vi "TLB Native Dynamic Events ver 0.05.vi"() -> ()   [LabVIEW 2018]
uses:
  Labview Training Phase 2/Enum Controls/States for Action Engine.ctl
  Type def/TLB event states.ctl
  Type def/TLB MHL States.ctl
  <vilib>/Studica/Studica Toolkit/Background/I2C Channel.ctl
  <vilib>/Studica/Studica Toolkit/NavX/NavX.lvlib
  <vilib>/myRIO/Common/Instrument Driver Framework/myRIO v1.0/AI/typedefs/AI Channels Enum.ctl
  <vilib>/myRIO/Common/Instrument Driver Framework/myRIO v1.0/AI/typedefs/AI Channels List.ctl
  <vilib>/Studica/Studica Toolkit/Background/Mxp Selection.ctl
  <vilib>/ptbypt/NI_PtbyPt.lvlib
panel:
  out "Yaw":dbl
  in  "NavX Zero Yaw":bool
  out "NavX Info Out":T2
  out "LinearAcceleration":T3
  out "Displacement":T4
  out "YRPHfH":T5
  in  "y":dbl=-1.2 format="%#_13g"
  out "Distance":T6
  in  "Return to IDLE":bool
  out "Sharp IR Distance":dbl
  out "Sharp IR Distance 2":dbl
  out "CM":fxp<+,64,16>
  out "Ultrasonic sensor":dbl format="%0.2f"
  out "Waveform Chart 3":dbl(graph)
  in  "xTargetSpeed":dbl
  in  "yTargetSpeed":dbl
  in  "wTargetSpeed":dbl
  out "Speed":T7
  in  "Reset Encoder 0":bool
  out "Action Queue Items":i32
  out "State Logic Queue Items":i32
  out "Action Queues items":string[](array[string])=["Hardware reset", "Software reset", ""]
  out "State logic":T8=enum."Task 2"
  out "Action State":string
  in  "Tasks Selector":string(combo)="Task 2"
  in  "Stop Queue":bool
  in  "Start Task":bool
  # "Test Programme written by Calvin Loke    Dated: 28 Aug 2019\nTest Programme revised by Dr Alex See   Dated 30 Aug 2019\n\nProgramme version:   TLB Native Dynamic Events ver 0.04b.vi"
  # "System Health Status Update"
  # "Sequence of Actions"
  # "Continuous (Repeated)"
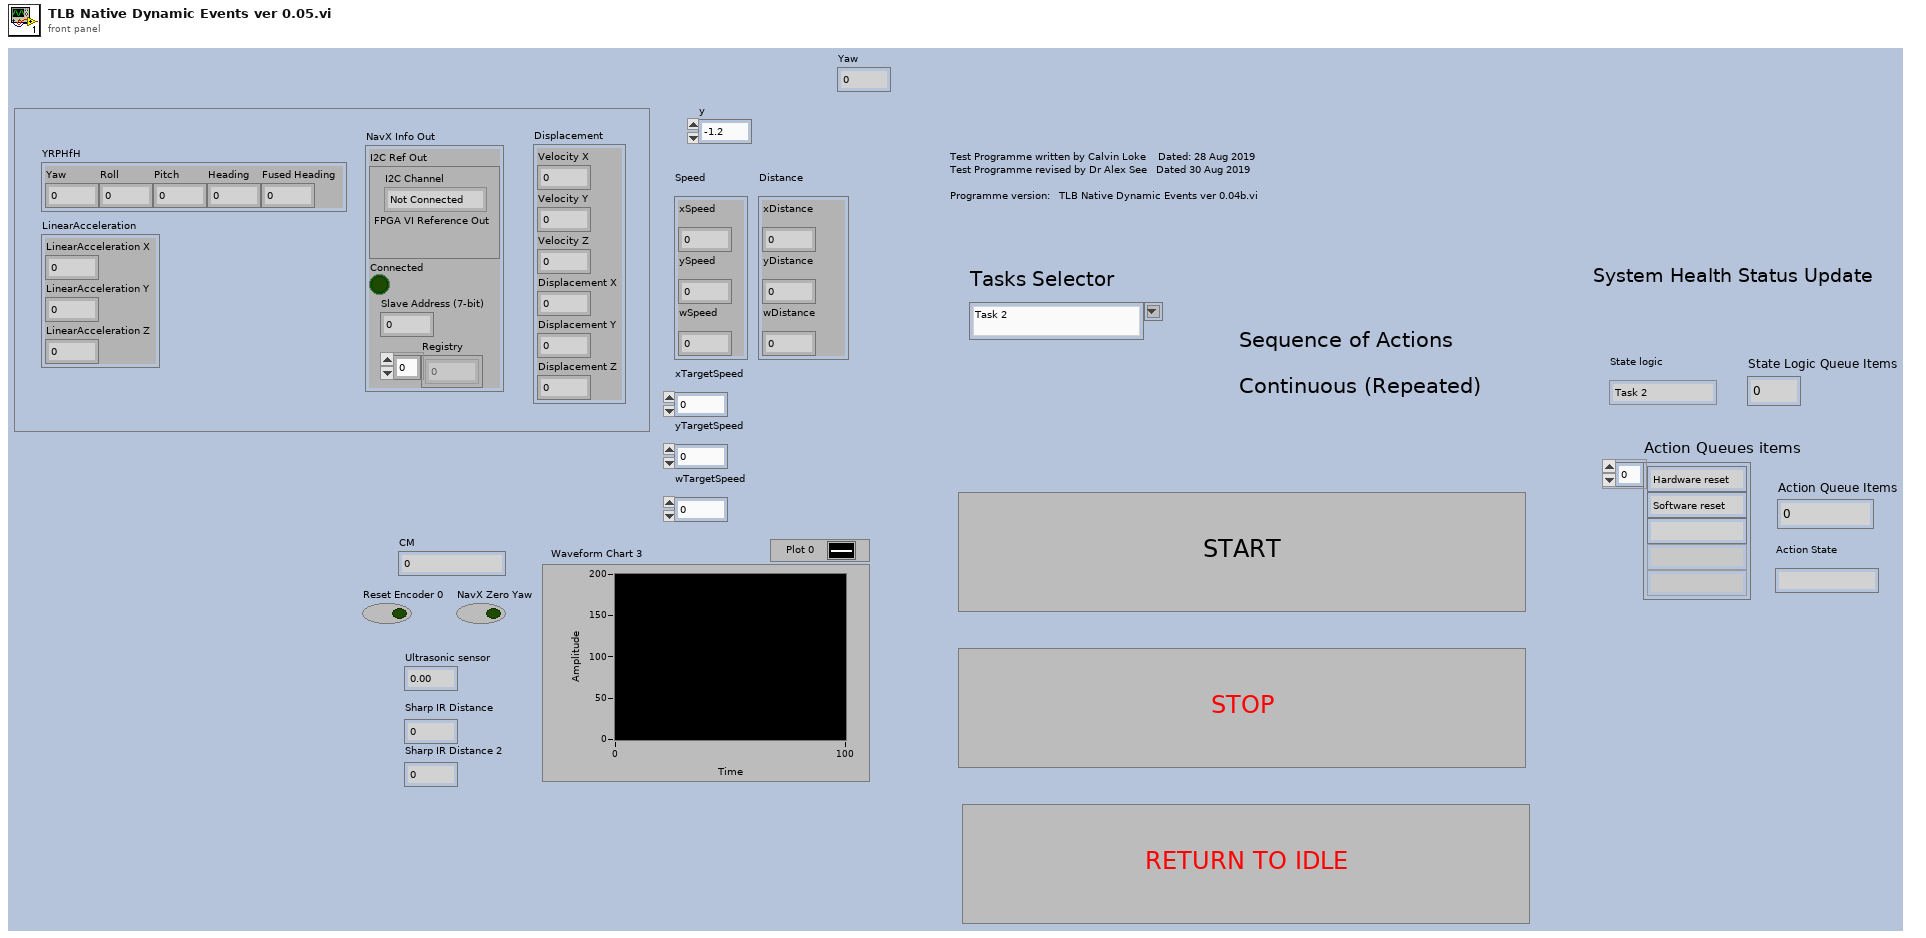
[diagram p1: front panel]
types:
  T1 = typedef "I2C Channel.ctl" = enum16{"Not Connected", "A", "B"}
  T2 = cluster{"I2C Ref Out":cluster{"I2C Channel":T1, "FPGA VI Reference Out":refnum<k20>}, "Connected":bool, "Slave Address (7-bit)":u8, "Registry":u8[]}
  T3 = cluster{"LinearAcceleration X":dbl, "LinearAcceleration Y":dbl, "LinearAcceleration Z":dbl}
  T4 = cluster{"Velocity X":dbl, "Velocity Y":dbl, "Velocity Z":dbl, "Displacement X":dbl, "Displacement Y":dbl, "Displacement Z":dbl}
  T5 = cluster{"Yaw":dbl, "Roll":dbl, "Pitch":dbl, "Heading":dbl, "Fused Heading":dbl}
  T6 = cluster{"xDistance":dbl, "yDistance":dbl, "wDistance":dbl}
  T7 = cluster{"xSpeed":dbl, "ySpeed":dbl, "wSpeed":dbl}
  T8 = typedef "TLB MHL States.ctl" = enum16{"None", "Startup", "Idle", "Processing", "Shutdown", "Reset", "Task 1", "Task 2", "Task 3", "Task 4", "Task 4a", "Task 4b", "Task 4c", "Task 4d", "Task 4e", "Task 4f", "Task 4g", "Task 4h", "Acquire image", "Wall follow mode", "Autodrive", "Autodrive a"}
  T9 = typedef "States for Action Engine.ctl" = enum16{"Initialize", "Write", "Read"}
  T10 = typedef "TLB event states.ctl" = enum16{"Start Sequence", "Exit", "Start Task 1", "Start Task 2", "Start Task 3", "Start Task 4", "Camera vision", "Wall follow mode", "Idle", "Start Drive Straight"}
  T11 = typedef "Mxp Selection.ctl" = enum16{"MXP A", "MXP B"}
  T12 = typedef "AI Channels List.ctl" = T13[]
  T13 = typedef "AI Channels Enum.ctl" = enum16{"Not Connected", "AudioIn/Left", "AudioIn/Right", "C/AI0", "C/AI1", "A/AI0", "A/AI1", "A/AI2", "A/AI3", "A/AI4", "A/AI5", "A/AI6", "A/AI7", "B/AI0", "B/AI1", "B/AI2", "B/AI3", "B/AI4", "B/AI5", "B/AI6", "B/AI7", "AI/AI0", "AI/AI1", "AI/AI2", "AI/AI3", "A/AI0 (DIFF)", "A/AI1 (DIFF)", "A/AI2 (DIFF)", "A/AI3 (DIFF)", "B/AI0 (DIFF)", "B/AI1 (DIFF)", "B/AI2 (DIFF)", "B/AI3 (DIFF)"}
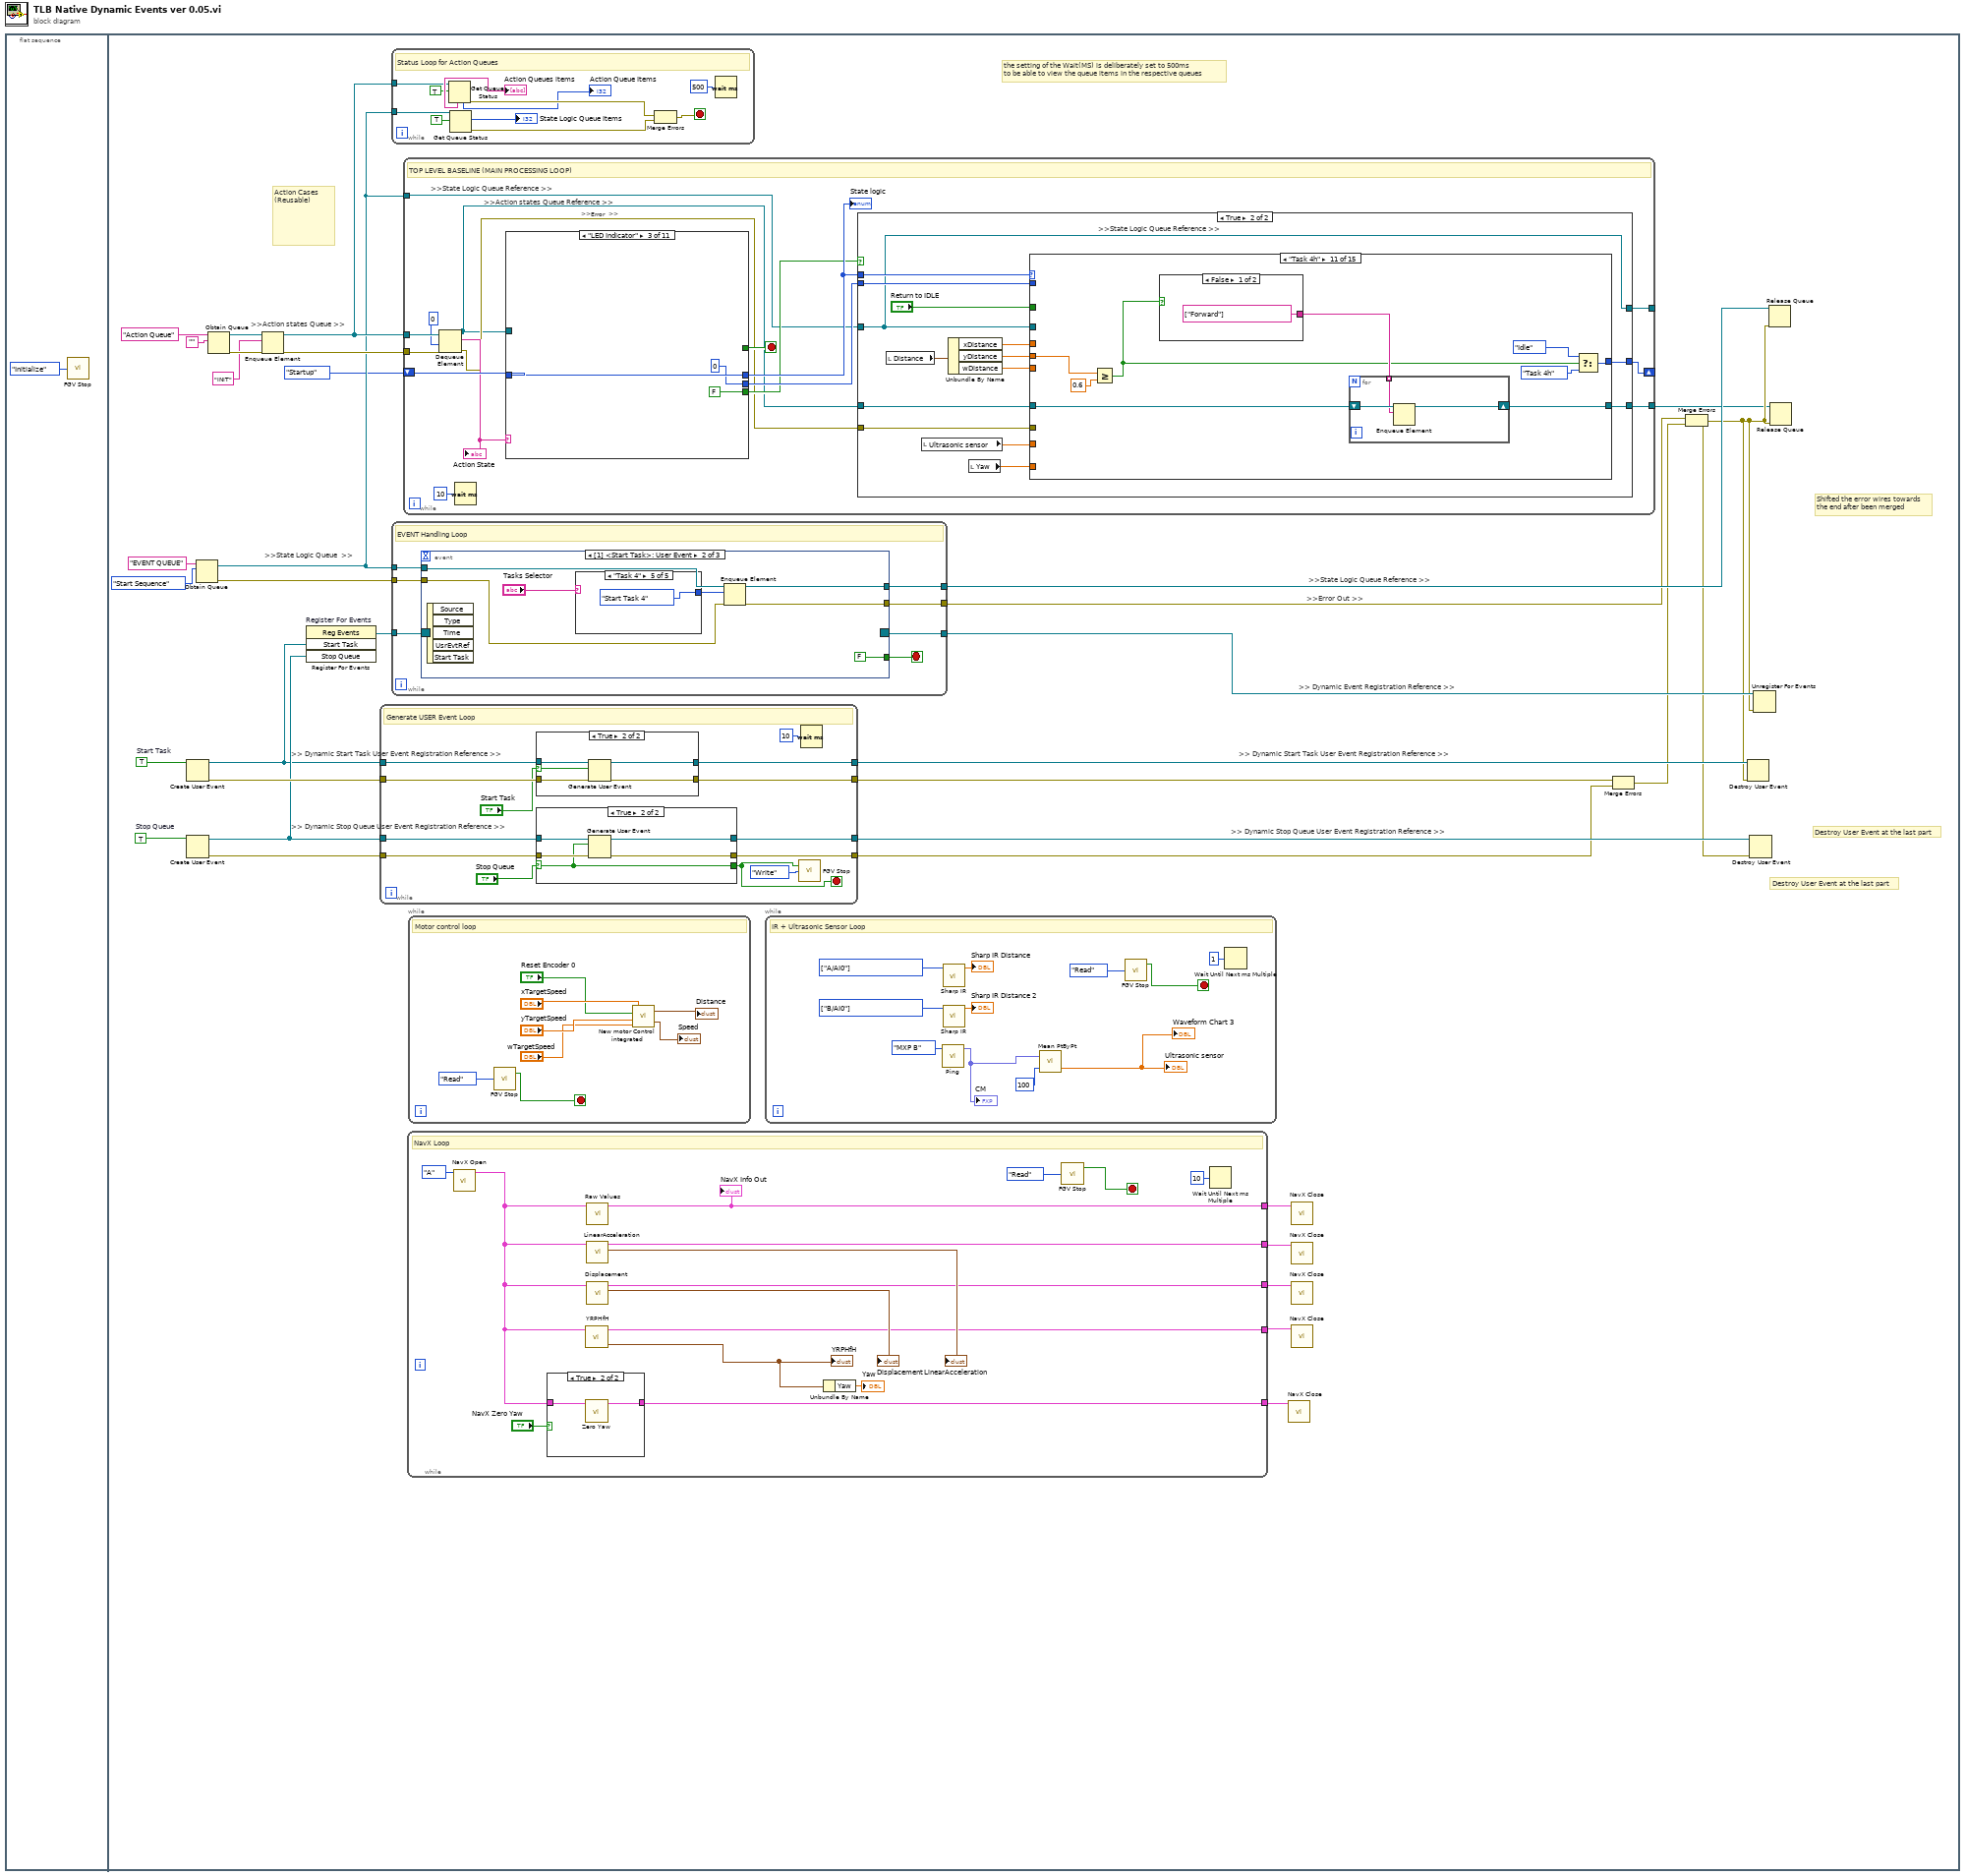
[diagram p0: block diagram]
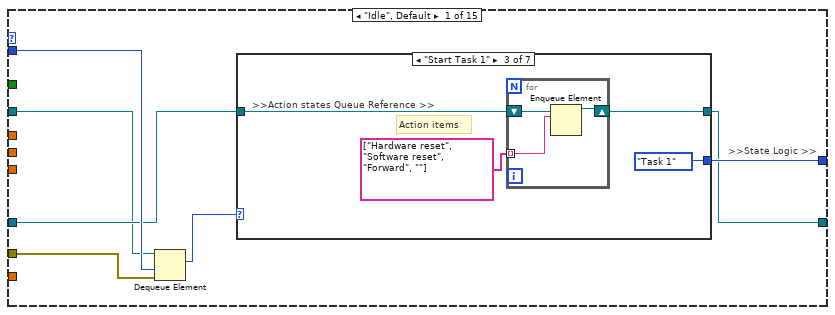
[diagram p4: hidden frame]
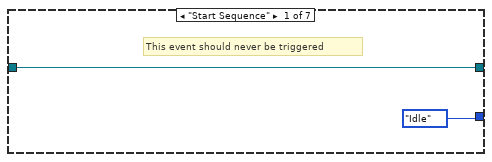
[diagram p5: hidden frame]
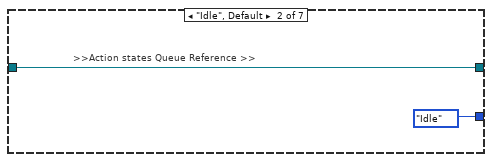
[diagram p6: hidden frame]
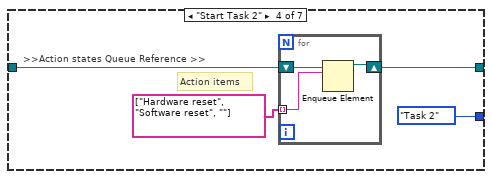
[diagram p7: hidden frame]
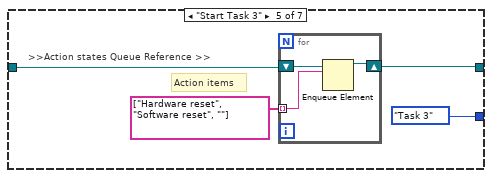
[diagram p8: hidden frame]
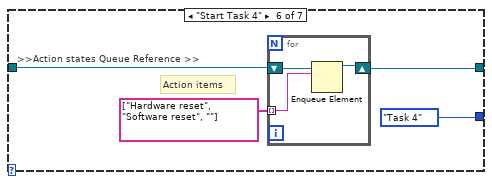
[diagram p9: hidden frame]
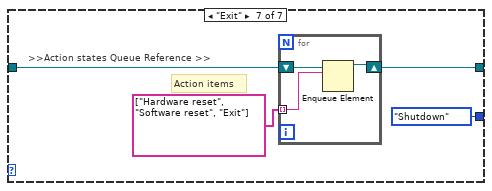
[diagram p10: hidden frame]
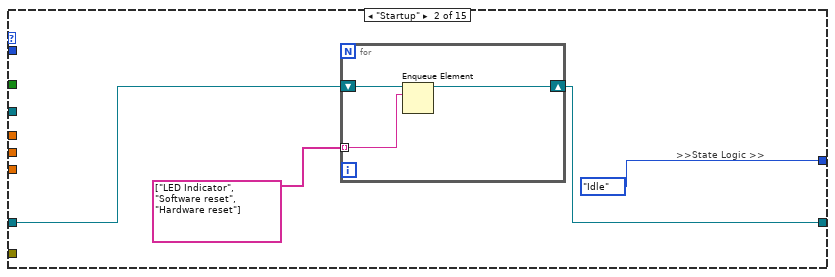
[diagram p11: hidden frame]
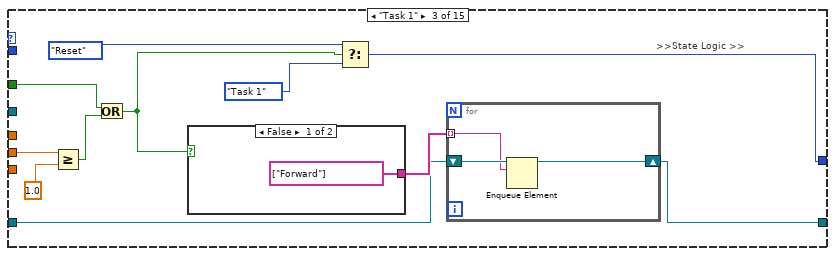
[diagram p12: hidden frame]
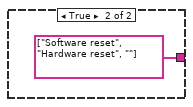
[diagram p13: hidden frame]
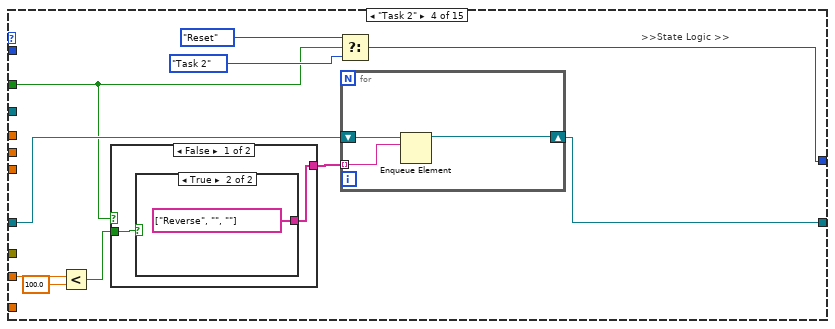
[diagram p14: hidden frame]
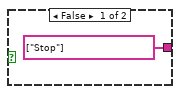
[diagram p15: hidden frame]
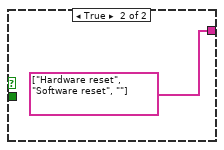
[diagram p16: hidden frame]
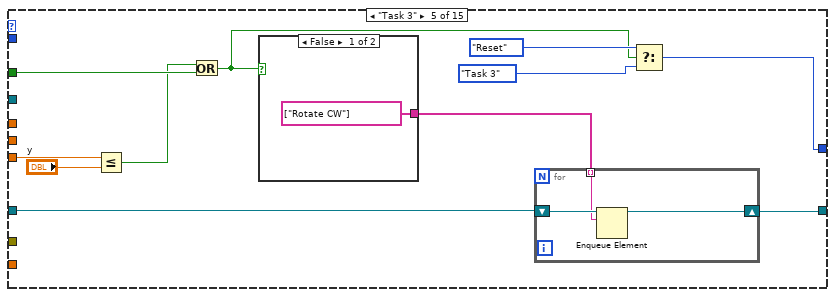
[diagram p17: hidden frame]
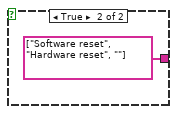
[diagram p18: hidden frame]
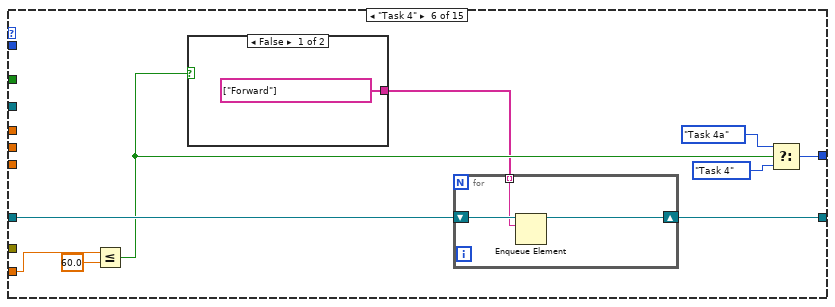
[diagram p19: hidden frame]
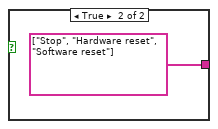
[diagram p20: hidden frame]
diagram:
  n1 = flat-sequence {
    frame #0 {
      n2 = call "FGV Stop.vi"("Init/Read/Write State"=States_for_Action_Engine."Initialize") -> ()  [unwired: 2 in, 2 out]
    }
    frame #1 {
      w35 = TRUE  # Stop Queue
      w34 = TRUE  # Start Task
      # "the setting of the Wait(MS) is deliberately set to 500ms\nto be able to view the queue items in the respective queues"
      # "Action Cases\n(Reusable)"
      # ">>Error Out >>"
      # ">> Dynamic Stop Queue User Event Registration Reference >>"
      # ">> Dynamic Start Task User Event Registration Reference >>"
      # ">> Dynamic Stop Queue User Event Registration Reference >>"
      # ">> Dynamic Start Task User Event Registration Reference >>"
      # ">> Dynamic Event Registration Reference >>"
      # ">>Action states Queue >>"
      # ">>State Logic Queue  >>"
      # ">>State Logic Queue Reference >>"
      # "Destroy User Event at the last part"
      # "Destroy User Event at the last part"
      # "Shifted the error wires towards\nthe end after been merged"
      n3 = Create User Event(user event datatype=w34) -> (user event=w26:refnum<user-event>, error out=w31:errorcluster)  [unwired: 1 in]
      n4 = Create User Event(user event datatype=w35) -> (user event=w27:refnum<user-event>, error out=w30:errorcluster)  [unwired: 1 in]
      n5 = Obtain Queue(name (unnamed)="EVENT QUEUE", element data type=TLB_event_states."Start Sequence" ("Enum")) -> (queue out=w11:refnum<queue>, error out=w17:errorcluster)  [unwired: 3 in, 1 out]
      n6 = Obtain Queue(name (unnamed)="Action Queue", element data type="") -> (queue out=w20:refnum<queue>, error out=w16:errorcluster)  [unwired: 3 in, 1 out]
      n7 = Enqueue Element(queue=w20, element="INIT", error in (no error)=w16) -> (queue out=w12:refnum<queue>, error out=w15:errorcluster)  [unwired: 1 in, 1 out]
      n8 = register-events "Register For Events"(w26, w27) -> (reference out=w25:refnum<event-registration>)  [unwired: 2 in, 1 out]
      n9 = while {
        tunnel: w26 -> [w424]
        tunnel: w27 -> [w423]
        tunnel: [w422] -> w33
        tunnel: [w421] -> w32
        tunnel: w31 -> [w420]
        tunnel: [w419] -> w29
        tunnel: w30 -> [w418]
        tunnel: [w417] -> w28
        stop <- w413 stop-if-true
        # "Generate USER Event Loop"
        n10 = case shown="True" "Start Task" {
          selector: "Start Task" -> [_ w436]
          tunnel: w424 -> [w435 w440]
          tunnel: [w435 w439] -> w421
          tunnel: w420 -> [w434 w438]
          tunnel: [w434 w437] -> w419
          frame False {
          }
          frame True {
            n11 = Generate User Event(user event=w440, event data cluster=w436, error in=w438) -> (user event out=w439:refnum<user-event>, error out=w437:errorcluster)  [unwired: 1 in]
          }
        }
        n12 = case shown="True" "Stop Queue" {
          selector: "Stop Queue" -> [_ w429]
          tunnel: w423 -> [w428 w433]
          tunnel: [w428 w432] -> w422
          tunnel: w418 -> [w427 w431]
          tunnel: [w427 w430] -> w417
          tunnel: [FALSE w429] -> w413
          frame False {
          }
          frame True {
            n13 = Generate User Event(user event=w433, event data cluster=w429, error in=w431) -> (user event out=w432:refnum<user-event>, error out=w430:errorcluster)  [unwired: 1 in]
          }
        }
        n14 = call "FGV Stop.vi"("Init/Read/Write State"=States_for_Action_Engine."Write", "Input Node"=w413) -> ()  [unwired: 1 in, 2 out]
        n15 = Wait (ms)(milliseconds to wait=u32 10) -> ()  [unwired: 1 out]
      }
      n16 = while {
        tunnel: w12 -> [w81]
        tunnel: w11 -> [w78]
        stop <- w75 stop-if-true
        # "Status Loop for Action Queues"
        n17 = Get Queue Status(queue=w81, return elements? (F)=TRUE) -> (error out=w77:errorcluster, # elements in queue=→"Action Queue Items":i32, elements=→"Action Queues items":string[])  [unwired: 1 in, 5 out]
        n18 = Get Queue Status(queue=w78, return elements? (F)=TRUE) -> (# pending remove=→"State Logic Queue Items":i32, error out=w76:errorcluster)  [unwired: 1 in, 6 out]
        n19 = Merge Errors(w77, w76) -> (w75:errorcluster)
        n20 = Wait (ms)(milliseconds to wait=u32 500) -> ()  [unwired: 1 out]
      }
      n21 = while {
        tunnel: w25 -> [w388]
        tunnel: [w387] -> w24
        tunnel: w11 -> [w385]
        tunnel: [w384] -> w23
        tunnel: w17 -> [w383]
        tunnel: [w382] -> w14
        stop <- w386 stop-if-true
        # "EVENT Handling Loop"
        n22 = event shown="[1] <Start Task>: User Event" {
          selector: w388 -> [_ _ _]
          dyn-events: [_ _ _] -> w387
          timeout: _ -> [_ _ _]
          tunnel: [FALSE FALSE w412] -> w386
          tunnel: w385 -> [w393 w400 w410]
          tunnel: [w392 w399 w411] -> w384
          tunnel: w383 -> [w390 w396 w408]
          tunnel: [w389 w395 w407] -> w382
          event Timeout {
            n23 = event-data() -> ()  [unwired: 1 in, 3 out]
            n24 = Enqueue Element(queue=w393, element=TLB_event_states."Idle" ("Enum"), error in (no error)=w390) -> (queue out=w392:refnum<queue>, error out=w389:errorcluster)  [unwired: 1 in, 1 out]
          }
          event User Event {
            n25 = event-data() -> ()  [unwired: 1 in, 5 out]
            n26 = case shown="\"Task 4\"" "Tasks Selector" {
              tunnel: [TLB_event_states."Idle" ("Enum") TLB_event_states."Start Task 1" ("Enum") TLB_event_states."Start Task 2" ("Enum") TLB_event_states."Start Task 3" ("Enum") TLB_event_states."Start Task 4" ("Enum")] -> w397
              frame Default {
              }
              frame "Task 1" {
              }
              frame "Task 2" {
              }
              frame "Task 3" {
              }
              frame "Task 4" {
              }
            }
            n27 = Enqueue Element(queue=w400, element=w397, error in (no error)=w396) -> (queue out=w399:refnum<queue>, error out=w395:errorcluster)  [unwired: 1 in, 1 out]
          }
          event User Event {
            n28 = event-data() -> ("Stop Queue"=w412:bool)  [unwired: 1 in, 4 out]
            n29 = Enqueue Element At Opposite End(queue=w410, element=TLB_event_states."Exit" ("Enum"), error in (no error)=w408) -> (queue out=w411:refnum<queue>, error out=w407:errorcluster)  [unwired: 1 in, 1 out]
          }
        }
      }
      n30 = while {
        tunnel: w11 -> [w86]
        shift-right: [w91] -> _
        shift-left: TLB_MHL_States."Startup" ("Enum") -> [w98]
        tunnel: w12 -> [w96]
        tunnel: w15 -> [w94]
        tunnel: [w93] -> _
        tunnel: [w92] -> w9
        stop <- w89 stop-if-true
        # ">>Error  >>"
        # ">>Action states Queue Reference >>"
        # ">>State Logic Queue Reference >>"
        # "TOP LEVEL BASELINE (MAIN PROCESSING LOOP)"
        n31 = Dequeue Element(queue=w96, timeout in ms (-1)=0, error in (no error)=w94) -> (queue out=w84:refnum<queue>, element=w95:string, error out=w85:errorcluster)  [unwired: 1 out]
        "Action State" <- w95
        n32 = Wait (ms)(milliseconds to wait=u32 10) -> ()  [unwired: 1 out]
        n33 = case shown="\"LED Indicator\"" w95 {
          tunnel: [w325 w330 w333 w339 w345 w354 w360 w366 w371 w377 TLB_MHL_States."Shutdown" ("Enum")] -> w97
          tunnel: w98 -> [w325 w330 w333 w339 w345 w354 w360 w366 w371 w377 _]
          tunnel: [w324 0 0 0 0 0 0 0 0 0 0] -> w90
          tunnel: [_ _ _ _ _ _ _ _ _ _ TRUE] -> w89
          tunnel: [TRUE FALSE FALSE FALSE FALSE FALSE FALSE FALSE FALSE FALSE FALSE] -> w88
          tunnel: w84 -> [_ _ _ _ _ _ _ _ _ _ _]
          frame "No action", Default {
            n34 = case shown="\"Idle\"" w325 {
              tunnel: [0 100] -> w324
              frame "Startup", Default {
              }
              frame "Idle" {
              }
            }
          }
          frame "Init" {
            # ">>State Logic  >>"
          }
          frame "LED Indicator" {
          }
          frame "Forward" {
            w335 = 0.0
            n35 = local write "NavX Zero Yaw"(FALSE ("NavX Zero Yaw")) -> ()
            n36 = local write "Reset Encoder 0"(FALSE ("Reset Encoder 0")) -> ()
            n37 = local write "wTargetSpeed"(w335) -> ()
            n38 = local write "yTargetSpeed"(0.5 ("yTargetSpeed")) -> ()
            n39 = local write "xTargetSpeed"(w335) -> ()
          }
          frame "Rotate CW" {
            w342 = 0.0
            n40 = local write "NavX Zero Yaw"(FALSE ("NavX Zero Yaw")) -> ()
            n41 = local write "Reset Encoder 0"(FALSE ("Reset Encoder 0")) -> ()
            n42 = local write "wTargetSpeed"(-0.15 ("yTargetSpeed")) -> ()
            n43 = local write "yTargetSpeed"(w342) -> ()
            n44 = local write "xTargetSpeed"(w342) -> ()
          }
          frame "Rotate ACW" {
            w351 = 0.0
            n45 = local write "NavX Zero Yaw"(FALSE ("NavX Zero Yaw")) -> ()
            n46 = local write "Reset Encoder 0"(FALSE ("Reset Encoder 0")) -> ()
            n47 = local write "wTargetSpeed"(0.15 ("yTargetSpeed")) -> ()
            n48 = local write "yTargetSpeed"(w351) -> ()
            n49 = local write "xTargetSpeed"(w351) -> ()
          }
          frame "Reverse" {
            w356 = 0.0
            n50 = local write "NavX Zero Yaw"(FALSE ("NavX Zero Yaw")) -> ()
            n51 = local write "Reset Encoder 0"(FALSE ("Reset Encoder 0")) -> ()
            n52 = local write "wTargetSpeed"(w356) -> ()
            n53 = local write "yTargetSpeed"(-0.3 ("yTargetSpeed")) -> ()
            n54 = local write "xTargetSpeed"(w356) -> ()
          }
          frame "Stop" {
            w363 = 0.0
            n55 = local write "NavX Zero Yaw"(FALSE ("NavX Zero Yaw")) -> ()
            n56 = local write "Reset Encoder 0"(FALSE ("Reset Encoder 0")) -> ()
            n57 = local write "wTargetSpeed"(w363) -> ()
            n58 = local write "yTargetSpeed"(w363) -> ()
            n59 = local write "xTargetSpeed"(w363) -> ()
          }
          frame "Software reset" {
            n60 = local write "NavX Zero Yaw"(FALSE ("NavX Zero Yaw")) -> ()
          }
          frame "Hardware reset" {
            w373 = 0.0
            n61 = local write "NavX Zero Yaw"(TRUE ("NavX Zero Yaw")) -> ()
            n62 = local write "Reset Encoder 0"(TRUE ("Reset Encoder 0")) -> ()
            n63 = local write "wTargetSpeed"(w373) -> ()
            n64 = local write "yTargetSpeed"(w373) -> ()
            n65 = local write "xTargetSpeed"(w373) -> ()
          }
          frame "Exit" {
          }
        }
        "State logic" <- w97
        n66 = case shown="True" w88 {
          tunnel: w97 -> [w101 w116]
          tunnel: w86 -> [w102 w110]
          tunnel: w84 -> [w100 w115]
          tunnel: [w102 w110] -> w93
          tunnel: [w100 w114] -> w92
          tunnel: [w101 w113] -> w91
          tunnel: w85 -> [_ w112]
          tunnel: w90 -> [_ w111]
          frame False {
          }
          frame True {
            # ">>State Logic Queue Reference >>"
            n67 = local read "Distance"() -> (w108:T6)
            n68 = local read "Ultrasonic sensor"() -> (w106:dbl)
            n69 = Unbundle By Name(w108) -> ("xDistance"=w104:dbl, "yDistance"=w107:dbl, "wDistance"=w105:dbl)
            n70 = local read "Yaw"() -> (w103:dbl)
            n71 = case shown="\"Task 4h\"" w116 {
              tunnel: w110 -> [w117 _ _ _ _ _ _ _ _ _ _ _ _ _ _]
              tunnel: w115 -> [w119 w164 w176 w191 w213 w224 w238 w251 w266 w278 w293 w306 w312 w315 w321]
              tunnel: [w118 w163 w175 w192 w212 w225 w237 w250 w265 w277 w292 w305 w312 w314 w321] -> w114
              tunnel: [w122 TLB_MHL_States."Idle" ("Enum") w178 w193 w209 w228 w240 w249 w267 w276 w291 TLB_MHL_States."Idle" ("Enum") TLB_MHL_States."Reset" ("Enum") TLB_MHL_States."Shutdown" ("Enum") TLB_MHL_States."Reset" ("Enum")] -> w113
              tunnel: w112 -> [w120 _ _ _ _ _ _ _ _ _ _ _ _ _ _]
              tunnel: w111 -> [w121 _ _ _ _ _ _ _ _ _ _ _ _ _ _]
              tunnel: "Return to IDLE" -> [_ _ w173 w188 w207 _ _ _ _ _ _ _ _ _ _]
              tunnel: w107 -> [_ _ w172 _ _ _ _ w248 _ w279 w290 _ _ _ _]
              tunnel: w106 -> [_ _ _ w190 _ w223 _ _ _ _ _ _ _ _ _]
              tunnel: w105 -> [_ _ _ _ w206 _ _ _ _ _ _ _ _ _ _]
              tunnel: w104 -> [_ _ _ _ _ _ _ _ _ _ _ _ _ _ _]
              tunnel: w103 -> [_ _ _ _ _ _ w236 _ w264 _ _ _ _ _ _]
              frame "Idle", Default {
                # ">>State Logic >>"
                n72 = Dequeue Element(queue=w117, timeout in ms (-1)=w121, error in (no error)=w120) -> (element=w123:T10)  [unwired: 3 out]
                n73 = case shown="\"Start Task 1\"" w123 {
                  tunnel: [TLB_MHL_States."Idle" ("Enum") TLB_MHL_States."Idle" ("Enum") TLB_MHL_States."Task 1" ("Enum") TLB_MHL_States."Task 2" ("Enum") TLB_MHL_States."Task 3" ("Enum") TLB_MHL_States."Task 4" ("Enum") TLB_MHL_States."Shutdown" ("Enum")] -> w122
                  tunnel: [w125 w126 w130 w135 w144 w150 w156] -> w118
                  tunnel: w119 -> [w125 w126 w128 w136 w145 w151 w157]
                  frame "Start Sequence" {
                    # "This event should never be triggered"
                  }
                  frame "Idle", Default {
                    # ">>Action states Queue Reference >>"
                  }
                  frame "Start Task 1" {
                    # ">>Action states Queue Reference >>"
                    # "Action items"
                    n74 = for {
                      shift-right: [w134] -> w130
                      shift-left: w128 -> [w133]
                      tunnel: string[] ["Hardware reset", "Software reset", "Forward", ""] -> [w132] mode=indexing
                      n75 = Enqueue Element(queue=w133, element=w132) -> (queue out=w134:refnum<queue>)  [unwired: 2 in, 2 out]
                    }
                  }
                  frame "Start Task 2" {
                    # ">>Action states Queue Reference >>"
                    # "Action items"
                    n76 = for {
                      shift-right: [w141] -> w135
                      shift-left: w136 -> [w140]
                      tunnel: string[] ["Hardware reset", "Software reset", ""] -> [w139] mode=indexing
                      n77 = Enqueue Element(queue=w140, element=w139) -> (queue out=w141:refnum<queue>)  [unwired: 2 in, 2 out]
                    }
                  }
                  frame "Start Task 3" {
                    # ">>Action states Queue Reference >>"
                    # "Action items"
                    n78 = for {
                      shift-right: [w148] -> w144
                      shift-left: w145 -> [w147]
                      tunnel: string[] ["Hardware reset", "Software reset", ""] -> [w146] mode=indexing
                      n79 = Enqueue Element(queue=w147, element=w146) -> (queue out=w148:refnum<queue>)  [unwired: 2 in, 2 out]
                    }
                  }
                  frame "Start Task 4" {
                    # ">>Action states Queue Reference >>"
                    # "Action items"
                    n80 = for {
                      shift-right: [w155] -> w150
                      shift-left: w151 -> [w154]
                      tunnel: string[] ["Hardware reset", "Software reset", ""] -> [w153] mode=indexing
                      n81 = Enqueue Element(queue=w154, element=w153) -> (queue out=w155:refnum<queue>)  [unwired: 2 in, 2 out]
                    }
                  }
                  frame "Exit" {
                    # ">>Action states Queue Reference >>"
                    # "Action items"
                    n82 = for {
                      shift-right: [w162] -> w156
                      shift-left: w157 -> [w161]
                      tunnel: string[] ["Hardware reset", "Software reset", "Exit"] -> [w160] mode=indexing
                      n83 = Enqueue Element(queue=w161, element=w160) -> (queue out=w162:refnum<queue>)  [unwired: 2 in, 2 out]
                    }
                  }
                }
              }
              frame "Startup" {
                # ">>State Logic >>"
                n84 = for {
                  shift-right: [w168] -> w163
                  shift-left: w164 -> [w169]
                  tunnel: string[] ["LED Indicator", "Software reset", "Hardware reset"] -> [w167] mode=indexing
                  n85 = Enqueue Element(queue=w169, element=w167) -> (queue out=w168:refnum<queue>)  [unwired: 2 in, 2 out]
                }
              }
              frame "Task 1" {
                # ">>State Logic >>"
                n86 = Greater Or Equal?(x=w172, y=1.0) -> (x >= y?=w170:bool)
                n87 = Or(x=w173, y=w170) -> (x .or. y?=w174:bool)
                n88 = case shown="False" w174 {
                  tunnel: [string[] ["Forward"] string[] ["Software reset", "Hardware reset", ""]] -> w177
                  frame False {
                  }
                  frame True {
                  }
                }
                n89 = Select(t=TLB_MHL_States."Reset" ("Enum"), s=w174, f=TLB_MHL_States."Task 1" ("Enum")) -> (s? t:f=w178:T8)
                n90 = for {
                  shift-right: [w184] -> w175
                  shift-left: w176 -> [w185]
                  tunnel: w177 -> [w183] mode=indexing
                  n91 = Enqueue Element(queue=w185, element=w183) -> (queue out=w184:refnum<queue>)  [unwired: 2 in, 2 out]
                }
              }
              frame "Task 2" {
                # ">>State Logic >>"
                n92 = Less?(x=w190, y=100.0) -> (x < y?=w186:bool)
                n93 = case shown="False" w188 {
                  tunnel: [w196 string[] ["Hardware reset", "Software reset", ""]] -> w187
                  tunnel: w186 -> [w197 _]
                  frame False {
                    n94 = case shown="True" w197 {
                      tunnel: [string[] ["Stop"] string[] ["Reverse", "", ""]] -> w196
                      frame False {
                      }
                      frame True {
                      }
                    }
                  }
                  frame True {
                  }
                }
                n95 = Select(t=TLB_MHL_States."Reset" ("Enum"), s=w188, f=TLB_MHL_States."Task 2" ("Enum")) -> (s? t:f=w193:T8)
                n96 = for {
                  shift-right: [w202] -> w192
                  shift-left: w191 -> [w203]
                  tunnel: w187 -> [w201] mode=indexing
                  n97 = Enqueue Element(queue=w203, element=w201) -> (queue out=w202:refnum<queue>)  [unwired: 2 in, 2 out]
                }
              }
              frame "Task 3" {
                n98 = Less Or Equal?(x=w206, y="y") -> (x <= y?=w204:bool)
                n99 = Or(x=w204, y=w207) -> (x .or. y?=w208:bool)
                n100 = case shown="False" w208 {
                  tunnel: [string[] ["Rotate CW"] string[] ["Software reset", "Hardware reset", ""]] -> w214
                  frame False {
                  }
                  frame True {
                  }
                }
                n101 = for {
                  shift-right: [w216] -> w212
                  shift-left: w213 -> [w217]
                  tunnel: w214 -> [w215] mode=indexing
                  n102 = Enqueue Element(queue=w217, element=w215) -> (queue out=w216:refnum<queue>)  [unwired: 2 in, 2 out]
                }
                n103 = Select(t=TLB_MHL_States."Reset" ("Enum"), s=w208, f=TLB_MHL_States."Task 3" ("Enum")) -> (s? t:f=w209:T8)
              }
              frame "Task 4" {
                n104 = Less Or Equal?(x=w223, y=60.0) -> (x <= y?=w221:bool)
                n105 = case shown="False" w221 {
                  tunnel: [string[] ["Forward"] string[] ["Stop", "Hardware reset", "Software reset"]] -> w220
                  frame False {
                  }
                  frame True {
                  }
                }
                n106 = for {
                  shift-right: [w232] -> w225
                  shift-left: w224 -> [w233]
                  tunnel: w220 -> [w231] mode=indexing
                  n107 = Enqueue Element(queue=w233, element=w231) -> (queue out=w232:refnum<queue>)  [unwired: 2 in, 2 out]
                }
                n108 = Select(t=TLB_MHL_States."Task 4a" ("Enum"), s=w221, f=TLB_MHL_States."Task 4" ("Enum")) -> (s? t:f=w228:T8)
              }
              frame "Task 4a" {
                n109 = Greater Or Equal?(x=w236, y=85.0) -> (x >= y?=w234:bool)
                n110 = case shown="False" w234 {
                  tunnel: [string[] ["Rotate CW"] string[] ["Stop", "Hardware reset", "Software reset"]] -> w239
                  frame False {
                  }
                  frame True {
                  }
                }
                n111 = for {
                  shift-right: [w246] -> w237
                  shift-left: w238 -> [w247]
                  tunnel: w239 -> [w245] mode=indexing
                  n112 = Enqueue Element(queue=w247, element=w245) -> (queue out=w246:refnum<queue>)  [unwired: 2 in, 2 out]
                }
                n113 = Select(t=TLB_MHL_States."Task 4b" ("Enum"), s=w234, f=TLB_MHL_States."Task 4a" ("Enum")) -> (s? t:f=w240:T8)
              }
              frame "Task 4b" {
                n114 = Greater Or Equal?(x=w248, y=0.15) -> (x >= y?=w252:bool)
                n115 = case shown="False" w252 {
                  tunnel: [string[] ["Forward"] string[] ["Stop", "Hardware reset", "Software reset"]] -> w253
                  frame False {
                  }
                  frame True {
                  }
                }
                n116 = for {
                  shift-right: [w260] -> w250
                  shift-left: w251 -> [w261]
                  tunnel: w253 -> [w259] mode=indexing
                  n117 = Enqueue Element(queue=w261, element=w259) -> (queue out=w260:refnum<queue>)  [unwired: 2 in, 2 out]
                }
                n118 = Select(t=TLB_MHL_States."Task 4c" ("Enum"), s=w252, f=TLB_MHL_States."Task 4b" ("Enum")) -> (s? t:f=w249:T8)
              }
              frame "Task 4c" {
                n119 = Less Or Equal?(x=w264, y=-85.0) -> (x <= y?=w262:bool)
                n120 = case shown="False" w262 {
                  tunnel: [string[] ["Rotate ACW"] string[] ["Stop", "Hardware reset", "Software reset"]] -> w268
                  frame False {
                  }
                  frame True {
                  }
                }
                n121 = for {
                  shift-right: [w274] -> w265
                  shift-left: w266 -> [w275]
                  tunnel: w268 -> [w273] mode=indexing
                  n122 = Enqueue Element(queue=w275, element=w273) -> (queue out=w274:refnum<queue>)  [unwired: 2 in, 2 out]
                }
                n123 = Select(t=TLB_MHL_States."Task 4d" ("Enum"), s=w262, f=TLB_MHL_States."Task 4c" ("Enum")) -> (s? t:f=w267:T8)
              }
              frame "Task 4d" {
                n124 = Greater Or Equal?(x=w279, y=0.8) -> (x >= y?=w280:bool)
                n125 = case shown="False" w280 {
                  tunnel: [string[] ["Forward"] string[] ["Stop", "Hardware reset", "Software reset"]] -> w281
                  frame False {
                  }
                  frame True {
                  }
                }
                n126 = for {
                  shift-right: [w288] -> w277
                  shift-left: w278 -> [w289]
                  tunnel: w281 -> [w287] mode=indexing
                  n127 = Enqueue Element(queue=w289, element=w287) -> (queue out=w288:refnum<queue>)  [unwired: 2 in, 2 out]
                }
                n128 = Select(t=TLB_MHL_States."Task 4e" ("Enum"), s=w280, f=TLB_MHL_States."Task 4d" ("Enum")) -> (s? t:f=w276:T8)
              }
              frame "Task 4h" {
                n129 = Greater Or Equal?(x=w290, y=0.6) -> (x >= y?=w294:bool)
                n130 = case shown="False" w294 {
                  tunnel: [string[] ["Forward"] string[] ["Stop", "Hardware reset", "Software reset"]] -> w295
                  frame False {
                  }
                  frame True {
                  }
                }
                n131 = for {
                  shift-right: [w302] -> w292
                  shift-left: w293 -> [w303]
                  tunnel: w295 -> [w301] mode=indexing
                  n132 = Enqueue Element(queue=w303, element=w301) -> (queue out=w302:refnum<queue>)  [unwired: 2 in, 2 out]
                }
                n133 = Select(t=TLB_MHL_States."Idle" ("Enum"), s=w294, f=TLB_MHL_States."Task 4h" ("Enum")) -> (s? t:f=w291:T8)
              }
              frame "Reset" {
                n134 = for {
                  shift-right: [w310] -> w305
                  shift-left: w306 -> [w311]
                  tunnel: string[] ["Software reset", "Hardware reset", ""] -> [w309] mode=indexing
                  n135 = Enqueue Element(queue=w311, element=w309) -> (queue out=w310:refnum<queue>)  [unwired: 2 in, 2 out]
                }
                n136 = Wait (ms)(milliseconds to wait=u32 250) -> ()  [unwired: 1 out]
              }
              frame "Processing" {
              }
              frame "Shutdown" {
                # ">>State Logic >>"
                n137 = for {
                  shift-right: [w319] -> w314
                  shift-left: w315 -> [w320]
                  tunnel: string[] ["Software reset", "Hardware reset", "Exit"] -> [w318] mode=indexing
                  n138 = Enqueue Element(queue=w320, element=w318) -> (queue out=w319:refnum<queue>)  [unwired: 2 in, 2 out]
                }
              }
              frame "None" {
              }
            }
          }
        }
      }
      n139 = while {
        tunnel: [w58] -> w7
        tunnel: [w55] -> w6
        tunnel: [w54] -> w4
        tunnel: [w53] -> w5
        tunnel: [w50] -> w3
        stop <- w60 stop-if-true
        # "NavX Loop"
        n140 = call <vilib>:"NavX Open.vi"("I2C Channel"=I2C_Channel."A") -> ("NavX Info"=w51:T2)  [unwired: 9 in, 1 out]
        n141 = case shown="True" "NavX Zero Yaw" {
          tunnel: w51 -> [w62 w64]
          tunnel: [w62 w63] -> w50
          frame False {
          }
          frame True {
            n142 = call <vilib>:"Zero Yaw.vi"("NavX Info In"=w64) -> ("NavX Info Out"=w63:T2)  [unwired: 10 in]
          }
        }
        n143 = call <vilib>:"YRPHfH.vi"("NavX Info In"=w51) -> ("YRPHfH"=w48:T5, "NavX Info Out"=w54:T2)  [unwired: 3 in]
        "YRPHfH" <- w48
        n144 = call <vilib>:"Raw Values.vi"("NavX Info In"=w51) -> ("NavX Info Out"=w58:T2)  [unwired: 8 in, 1 out]
        "NavX Info Out" <- w58
        n145 = call <vilib>:"LinearAcceleration.vi"("NavX Info In"=w51) -> ("LinearAcceleration"=→"LinearAcceleration":T3, "NavX Info Out"=w55:T2)  [unwired: 9 in]
        n146 = call <vilib>:"Displacement.vi"("NavX Info In"=w51) -> ("Displacement"=→"Displacement":T4, "NavX Info Out"=w53:T2)  [unwired: 9 in]
        n147 = Unbundle By Name(w48) -> ("Yaw"=→"Yaw":dbl)
        n148 = call "FGV Stop.vi"("Init/Read/Write State"=States_for_Action_Engine."Read") -> ("Output node"=w60:bool)  [unwired: 2 in, 1 out]
        n149 = Wait Until Next ms Multiple(millisecond multiple=u32 10) -> ()  [unwired: 1 out]
      }
      n150 = while {
        stop <- w71 stop-if-true
        # "Motor control loop"
        n151 = call "FGV Stop.vi"("Init/Read/Write State"=States_for_Action_Engine."Read") -> ("Output node"=w71:bool)  [unwired: 2 in, 1 out]
        n152 = call "New motor Control integrated.vi"("wTargetSpeed"="wTargetSpeed", "yTargetSpeed"="yTargetSpeed", "xTargetSpeed"="Reset Encoder 0", "Reset Encoders"="xTargetSpeed") -> ("Speed"=→"Speed":T7, "Distance"=→"Distance":T6)
      }
      n153 = while {
        stop <- w40 stop-if-true
        w45 = T12 [enum."B/AI0"] items=["Not Connected", "AudioIn/Left", "AudioIn/Right", "C/AI0", "C/AI1", "A/AI0", "A/AI1", "A/AI2", "A/AI3", "A/AI4", "A/AI5", "A/AI6", "A/AI7", "B/AI0", "B/AI1", "B/AI2", "B/AI3", "B/AI4", "B/AI5", "B/AI6", "B/AI7", "AI/AI0", "AI/AI1", "AI/AI2", "AI/AI3", "A/AI0 (DIFF)", "A/AI1 (DIFF)", "A/AI2 (DIFF)", "A/AI3 (DIFF)", "B/AI0 (DIFF)", "B/AI1 (DIFF)", "B/AI2 (DIFF)", "B/AI3 (DIFF)"] ("AI Channel")
        w46 = T12 [enum."A/AI0"] items=["Not Connected", "AudioIn/Left", "AudioIn/Right", "C/AI0", "C/AI1", "A/AI0", "A/AI1", "A/AI2", "A/AI3", "A/AI4", "A/AI5", "A/AI6", "A/AI7", "B/AI0", "B/AI1", "B/AI2", "B/AI3", "B/AI4", "B/AI5", "B/AI6", "B/AI7", "AI/AI0", "AI/AI1", "AI/AI2", "AI/AI3", "A/AI0 (DIFF)", "A/AI1 (DIFF)", "A/AI2 (DIFF)", "A/AI3 (DIFF)", "B/AI0 (DIFF)", "B/AI1 (DIFF)", "B/AI2 (DIFF)", "B/AI3 (DIFF)"] ("AI Channel")
        # "IR + Ultrasonic Sensor Loop"
        n154 = call <vilib>:"Ping.vi"("Mxp Side"=Mxp_Selection."MXP B") -> ("CM"=w36:fxp<+,64,16>)  [unwired: 8 in, 2 out]
        "CM" <- w36
        n155 = call <vilib>:"Sharp IR.vi"("AI Channel"=w46) -> ("Sharp IR Distance"=→"Sharp IR Distance":dbl)  [unwired: 8 in, 2 out]
        n156 = call <vilib>:"Sharp IR.vi"("AI Channel"=w45) -> ("Sharp IR Distance"=→"Sharp IR Distance 2":dbl)  [unwired: 8 in, 2 out]
        n157 = call <vilib>:"Mean PtByPt.vi"("x"=w36, "sample length"=100) -> ("mean"=→"Ultrasonic sensor" →"Waveform Chart 3":dbl)  [unwired: 2 in, 1 out]
        n158 = call "FGV Stop.vi"("Init/Read/Write State"=States_for_Action_Engine."Read") -> ("Output node"=w40:bool)  [unwired: 2 in, 1 out]
        n159 = Wait Until Next ms Multiple(millisecond multiple=u32 1) -> ()  [unwired: 1 out]
      }
      n160 = call <vilib>:"NavX Close.vi"("NavX Info In"=w3) -> ()  [unwired: 10 in, 1 out]
      n161 = call <vilib>:"NavX Close.vi"("NavX Info In"=w7) -> ()  [unwired: 10 in, 1 out]
      n162 = call <vilib>:"NavX Close.vi"("NavX Info In"=w6) -> ()  [unwired: 10 in, 1 out]
      n163 = call <vilib>:"NavX Close.vi"("NavX Info In"=w5) -> ()  [unwired: 10 in, 1 out]
      n164 = call <vilib>:"NavX Close.vi"("NavX Info In"=w4) -> ()  [unwired: 10 in, 1 out]
      n165 = Merge Errors "Merge Errors"(w29, w28) -> (w8:errorcluster)
      n166 = Merge Errors(w14, w8) -> (w10:errorcluster)
      n167 = Destroy User Event(user event=w32, error in=w10) -> ()  [unwired: 1 out]
      n168 = Destroy User Event(user event=w33, error in=w10) -> ()  [unwired: 1 out]
      n169 = Unregister For Events(event registration refnum=w24, error in=w10) -> ()  [unwired: 1 out]
      n170 = Release Queue(queue=w23, error in (no error)=w10) -> ()  [unwired: 1 in, 3 out]
      n171 = Release Queue(queue=w9, error in (no error)=w10) -> ()  [unwired: 1 in, 3 out]
    }
  }
